vi "NanotecSMCPDDriver.get limit switch polarity.vi"(0 "VISA resource name":refnum<visa-resource-name>, 1 "contollerID":i32=-1, 5 "error in (no error)":errorcluster) -> (14 "VISA resource name out":refnum<visa-resource-name>, 15 "contollerID out":i32=-1, 17 "normallyClosed":bool, 19 "error out":errorcluster)   [LabVIEW 2014, in "NanotecSMCPDDriver.lvlib"]
doc: "Gets the polarity of the limit switch."
uses:
  NanotecSMCPDDriver.lvlib
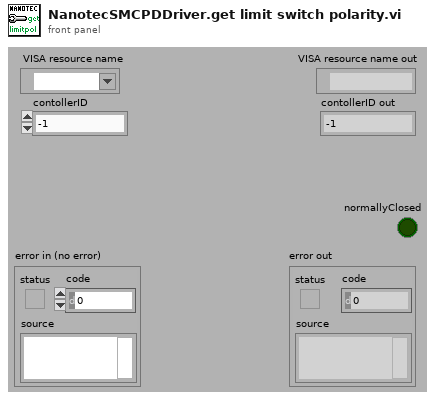
[diagram p1: front panel]
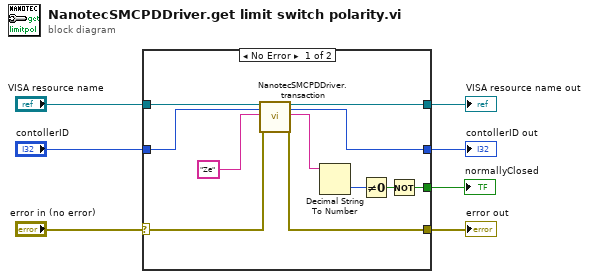
[diagram p0: block diagram]
diagram:
  n1 = case shown="No Error" "error in (no error)" {
    selector: "error in (no error)" -> [w11 w19]
    tunnel: [w14 w21] -> w7
    tunnel: [w12 w19] -> w6
    tunnel: "VISA resource name" -> [w18 w21]
    tunnel: "contollerID" -> [w16 w20]
    tunnel: [w15 w20] -> w3
    tunnel: [w8 _] -> w1
    frame No Error {
      n2 = call "NanotecSMCPDDriver.transaction.vi"("VISAresource"=w18, "contollerID"=w16, "commandString"="Ze", "error in (no error)"=w11) -> ("VISAresource out"=w14:refnum<visa-resource-name>, "contollerID out"=w15:i32, "response"=w13:string, "error out"=w12:errorcluster)  [unwired: 10 in, 2 out]
      n3 = Decimal String To Number(string=w13) -> (number=w10:i32)  [unwired: 2 in, 1 out]
      n4 = Not Equal To 0?(x=w10) -> (x != 0?=w9:bool)
      n5 = Not(x=w9) -> (.not. x?=w8:bool)
    }
    frame Error {
    }
  }
  "VISA resource name out" <- w7
  "error out" <- w6
  "contollerID out" <- w3
  "normallyClosed" <- w1
